vi "Write_All_Reg.vi"(0 "USB DAQ Address":i32 format="%x", 1 "Write I2C Address":u8 format="%x", 2 "Edited Register":bool[](array[boolean]), 3 "Slide Refnum":refnum<vi>, 4 "Index to Reg No":u8[](array[numeric]) format="%x", 5 "Register":u16[](array[numeric]) format="%x") -> (6 "Status":string="ERROR COMMUNICATING WITH DEVICE")   [LabVIEW 2011]
panel:
  out "Comm Error Flags":bool[](array[boolean])
  out "Status String Array":string[](array[string])
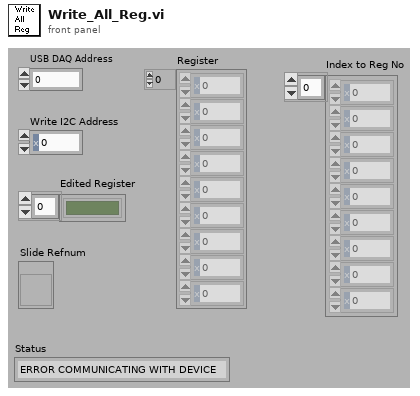
[diagram p1: front panel]
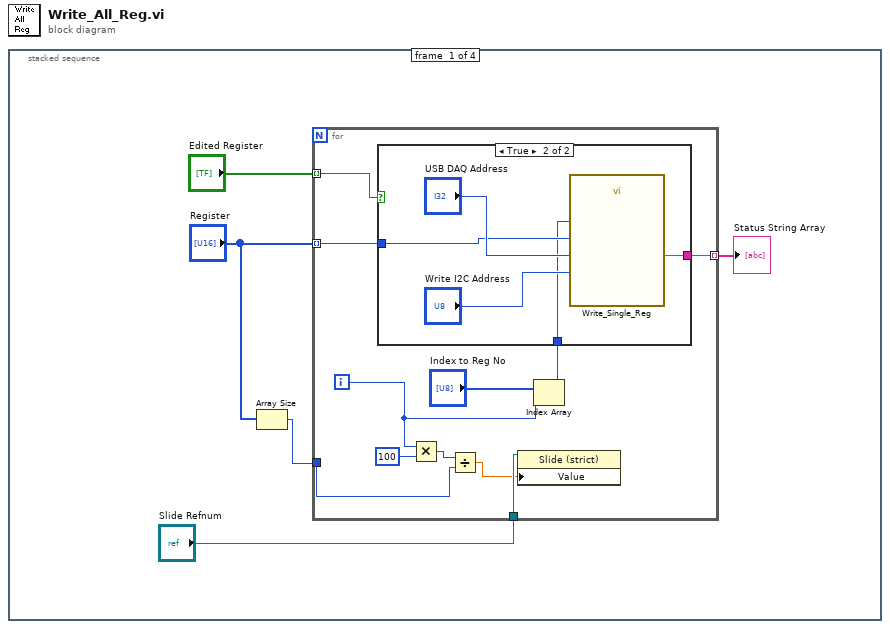
[diagram p0: block diagram]
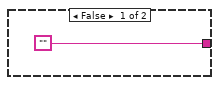
[diagram p2: hidden frame]
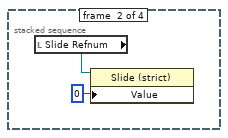
[diagram p3: hidden frame]
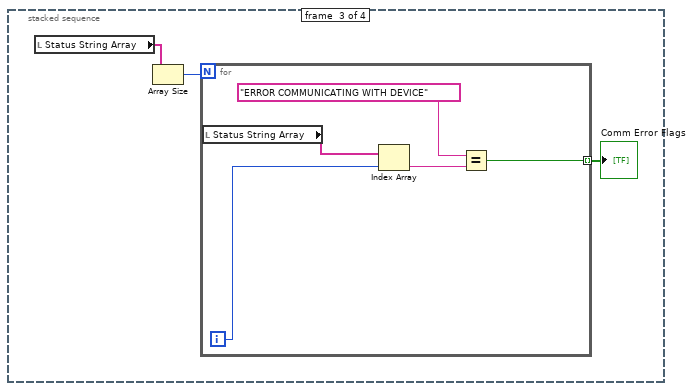
[diagram p4: hidden frame]
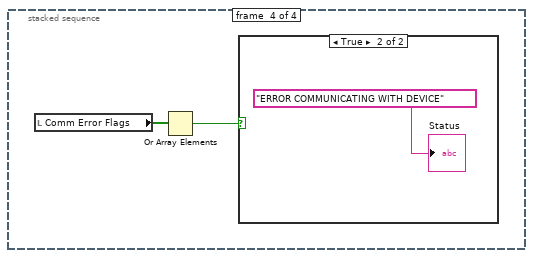
[diagram p5: hidden frame]
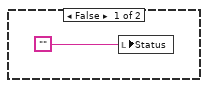
[diagram p6: hidden frame]
diagram:
  n1 = stacked-sequence {
    frame #0 {
      n2 = Array Size(array="Register") -> (size(s)=w2:i32)
      n3 = for {
        tunnel: "Edited Register" -> [w16] mode=indexing
        tunnel: "Register" -> [w10] mode=indexing
        tunnel: "Slide Refnum" -> [w14]
        tunnel: w2 -> [w11]
        tunnel: [w9] -> w5 mode=indexing
        i -> [w7]
        n4 = Multiply(x=w7, y=100) -> (x*y=w15:i32)
        n5 = Divide(x=w15, y=w11) -> (x/y=w13:dbl)
        n6 = property class="Slide (strict)"(reference=w14, "Value"=w13) -> ()  [unwired: 1 in, 2 out]
        n7 = Index Array(array="Index to Reg No", index=w7) -> (element=w6:u8)
        n8 = case shown="True" w16 {
          tunnel: w10 -> [_ w20]
          tunnel: ["" w19] -> w9
          tunnel: w6 -> [_ w18]
          frame False {
          }
          frame True {
            n9 = call "Write_Single_Reg.vi"("Reg No"=w18, "Write I2C Address"="Write I2C Address", "Reg Value"=w20, "USB DAQ Address"="USB DAQ Address") -> ("Status String"=w19:string)  [unwired: 1 in]
          }
        }
      }
      "Status String Array" <- w5
    }
    frame #1 {
      n10 = local read "Slide Refnum"() -> (w23:refnum<vi>)
      n11 = property class="Slide (strict)"(reference=w23, "Value"=u8 0) -> ()  [unwired: 1 in, 2 out]
    }
    frame #2 {
      n12 = local read "Status String Array"() -> (w25:string[])
      n13 = Array Size(array=w25) -> (size(s)=w27:i32)
      n14 = for {
        N: w27 -> [_]
        tunnel: [w30] -> w26 mode=indexing
        i -> [w32]
        n15 = local read "Status String Array"() -> (w29:string[])
        n16 = Index Array(array=w29, index=w32) -> (element=w28:string)
        n17 = Equal?(x="ERROR COMMUNICATING WITH DEVICE", y=w28) -> (x = y?=w30:bool)
      }
      "Comm Error Flags" <- w26
    }
    frame #3 {
      n18 = local read "Comm Error Flags"() -> (w33:bool[])
      n19 = Or Array Elements(Boolean array=w33) -> (logical OR=w34:bool)
      n20 = case shown="True" w34 {
        frame False {
          n21 = local write "Status"("") -> ()
        }
        frame True {
          "Status" <- "ERROR COMMUNICATING WITH DEVICE"
        }
      }
    }
  }
